vi "Read DoW.vi"(8 "error in (no error)":errorcluster, 11 "Daily in":refnum<class "Daily.lvclass">) -> (0 "error out":errorcluster, 2 "DoW":T1, 3 "Daily out":refnum<class "Daily.lvclass">)   [LabVIEW 2020, in "Daily.lvclass"]
uses:
  Daily.lvclass
  Daily.lvclass/Daily.ctl
  Daily DoW TYP.ctl
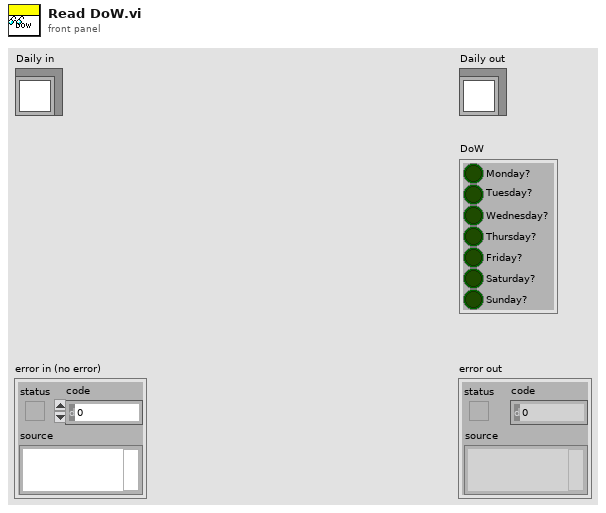
[diagram p1: front panel]
types:
  T1 = typedef "Daily.lvclass/Daily DoW TYP.ctl" = cluster{"Monday?":bool, "Tuesday?":bool, "Wednesday?":bool, "Thursday?":bool, "Friday?":bool, "Saturday?":bool, "Sunday?":bool}
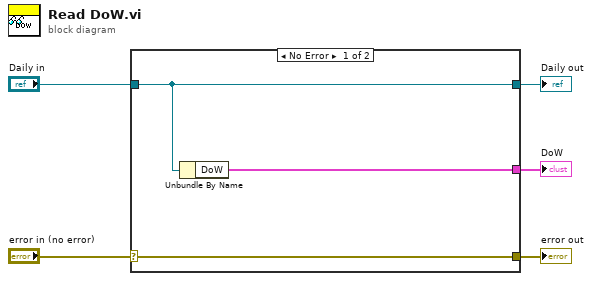
[diagram p0: block diagram]
diagram:
  n1 = case shown="No Error" "error in (no error)" {
    selector: "error in (no error)" -> [w8 w9]
    tunnel: [w8 w9] -> w4
    tunnel: [w7 w10] -> w2
    tunnel: "Daily in" -> [w7 w10]
    tunnel: [w6 _] -> w1
    frame No Error {
      n2 = Unbundle By Name(w7) -> ("DoW"=w6:T1)
    }
    frame Error {
    }
  }
  "error out" <- w4
  "Daily out" <- w2
  "DoW" <- w1
